vi "TPNT_CheckAlarmLevel.vi"(10 "testpoint In":T1={"name"="", "type"="", "algor"=[], "update_rate"=0.0, "Limits"={"Alarm Type"="", "Lower "=0.0, "Upper"=0.0, "Nominal"=0.0, "outrange"=FALSE, "Check"=TRUE, "latch"=FALSE, "level"=""}, "Samples"={"samples"=0, "counter"=0, "Values"=[], "Current Value"="", "filter"="", "precision"=2}, "next_update"=0, "Status"="", "monitor"=TRUE, "error"=FALSE, "Log"={"log"=FALSE, "file"=path "", "type"="", "format"="", "updaterate"=0.0, "nex_update"=0, "mode"=""}, "permissions"="", "ID"=""} {"Log"."updaterate" format="%.2f"; "Samples"."Values" format="%.2f"; "Samples"."samples" min=1 step=1; "Limits"."Nominal" format="%.2f"; "Limits"."Upper" format="%.2f"; "Limits"."Lower" format="%.2f"; "update_rate" format="%.2f"}) -> (2 "testpoint out":T1={"name"="", "type"="", "algor"=[], "update_rate"=0.0, "Limits"={"Alarm Type"="", "Lower "=0.0, "Upper"=0.0, "Nominal"=0.0, "outrange"=FALSE, "Check"=TRUE, "latch"=FALSE, "level"=""}, "Samples"={"samples"=0, "counter"=0, "Values"=[], "Current Value"="", "filter"="", "precision"=2}, "next_update"=0, "Status"="", "monitor"=TRUE, "error"=FALSE, "Log"={"log"=FALSE, "file"=path "", "type"="", "format"="", "updaterate"=0.0, "nex_update"=0, "mode"=""}, "permissions"="", "ID"=""} {"Log"."updaterate" format="%.2f"; "Samples"."Values" format="%.2f"; "Samples"."samples" min=1 step=1; "Limits"."Nominal" format="%.2f"; "Limits"."Upper" format="%.2f"; "Limits"."Lower" format="%.2f"; "update_rate" format="%.2f"})   [LabVIEW 2016]
uses:
  TPNT_TP.ctl
  TPNT_Limits.ctl
  TPNT_Samples.ctl
  TPNT_Log.ctl
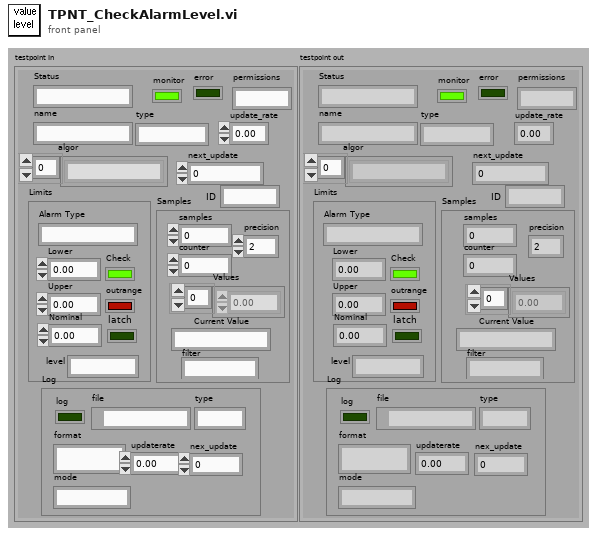
[diagram p1: front panel]
types:
  T1 = typedef "TPNT_TP.ctl" = cluster{"name":string, "type":string, "algor":string[], "update_rate":sgl, "Limits":T2, "Samples":T3, "next_update":u32, "Status":string, "monitor":bool, "error":bool, "Log":T4, "permissions":string, "ID":string}
  T2 = typedef "TPNT_Limits.ctl" = cluster{"Alarm Type":string, "Lower ":dbl, "Upper":dbl, "Nominal":dbl, "outrange":bool, "Check":bool, "latch":bool, "level":string}
  T3 = typedef "TPNT_Samples.ctl" = cluster{"samples":i32, "counter":i32, "Values":dbl[], "Current Value":string, "filter":string, "precision":u8}
  T4 = typedef "TPNT_Log.ctl" = cluster{"log":bool, "file":path, "type":string, "format":string, "updaterate":dbl, "nex_update":u32, "mode":string}
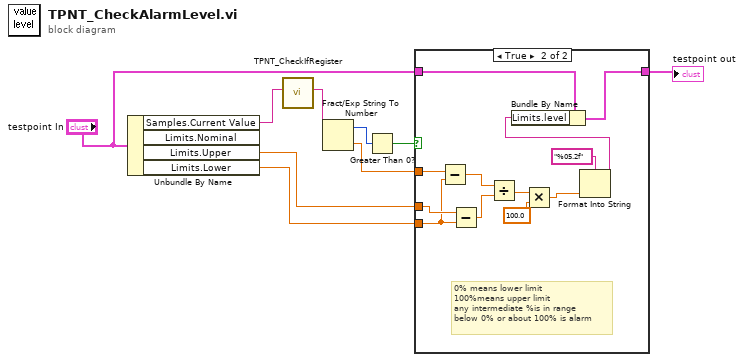
[diagram p0: block diagram]
diagram:
  n1 = Unbundle By Name("testpoint In") -> ("Samples.Current Value"=w8:string, "Limits.Upper"=w3:dbl, "Limits.Lower"=w2:dbl)  [unwired: 1 out]
  n2 = call "TPNT_CheckIfRegister.vi"("value in"=w8) -> ("value out"=w9:string)  [unwired: 10 out]
  n3 = Fract/Exp String To Number(string=w9) -> (offset past number=w1:i32, number=w6:dbl)  [unwired: 3 out]
  n4 = Greater Than 0?(x=w1) -> (x > 0?=w7:bool)
  n5 = case shown="True" w7 {
    tunnel: w6 -> [_ w19]
    tunnel: "testpoint In" -> [w10 w22]
    tunnel: [w10 w21] -> w4
    tunnel: w3 -> [_ w20]
    tunnel: w2 -> [_ w12]
    frame False {
    }
    frame True {
      # "0% means lower limit\n100%means upper limit\nany intermediate %is in range\nbelow 0% or about 100% is alarm"
      n6 = Subtract(x=w19, y=w12) -> (x-y=w18:dbl)
      n7 = Subtract(x=w20, y=w12) -> (x-y=w17:dbl)
      n8 = Divide(x=w18, y=w17) -> (x/y=w16:dbl)
      n9 = Multiply(x=w16, y=100.0) -> (x*y=w11:dbl)
      n10 = Format Into String(format string="%05.2f", w11) -> (resulting string=w13:string)  [unwired: 2 in, 1 out]
      n11 = Bundle By Name(cluster=w22, "Limits.level"=w13) -> (w21:T1)
    }
  }
  "testpoint out" <- w4
